vi "Unit Test.vi"() -> ()   [LabVIEW 2018, in "Optris PI.lvlib"]
uses:
  Optris PI/Optris PI.lvlib
  PPLs/Thermal Camera/Parent/Thermal Camera.lvlibp/Accessors/Area Coordinates.ctl
  <vilib>/Utility/miscctls.llb/LVPoint32TypeDef.ctl
  PPLs/Thermal Camera/Parent/Thermal Camera.lvlibp/Thermal Camera.lvclass
panel:
  out "Coords":T1
  out "Area Temps":dbl[][](array[numeric])
  out "Thermal Image":picture
  in  "Path":path=path "C:/RCVR_DATA/RCVRASSET/pic.bmp"
  in  "Cluster":T2={"X"=100, "X Offset"=50, "Y"=100, "Y Offset"=50}
  in  "Min":dbl=-40.0
  in  "Max":dbl=125.0
  in  "Get Thermal Image":bool
  out "error out":errorcluster
  in  "error in (no error)":errorcluster
  in  "Set Temp Range":bool
  in  "Stop":bool
  in  "Connect":bool
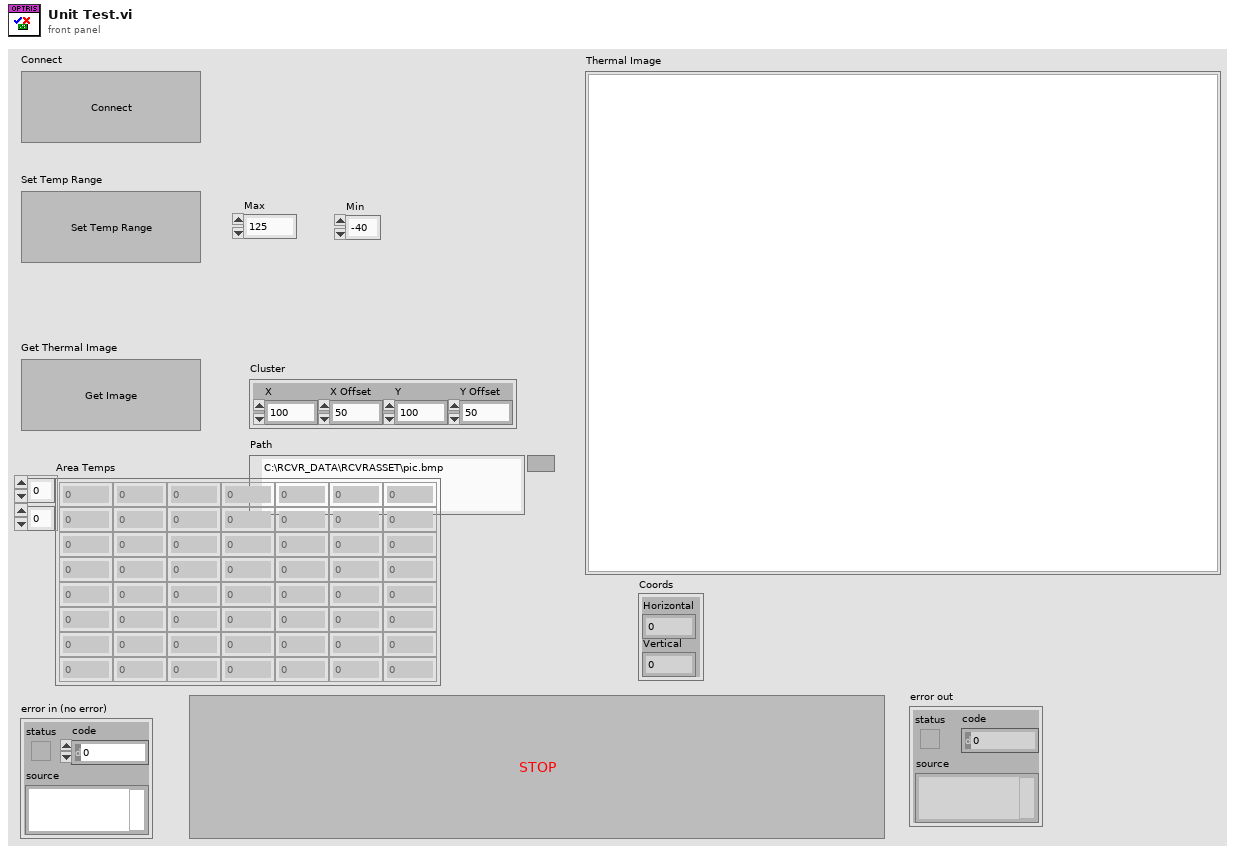
[diagram p1: front panel]
types:
  T1 = typedef "LVPoint32TypeDef.ctl" = cluster{"Horizontal":i32, "Vertical":i32}
  T2 = typedef "Thermal Camera.lvlibp/Thermal Camera.lvclass/Area Coordinates.ctl" = cluster{"X":i32, "X Offset":i32, "Y":i32, "Y Offset":i32}
  T3 = typedef "imagedata.ctl" = cluster{"image type":i32, "image depth":i32, "image":u8[], "mask":u8[], "colors":u32[], "Rectangle":cluster{"left":i16, "top":i16, "right":i16, "bottom":i16}}
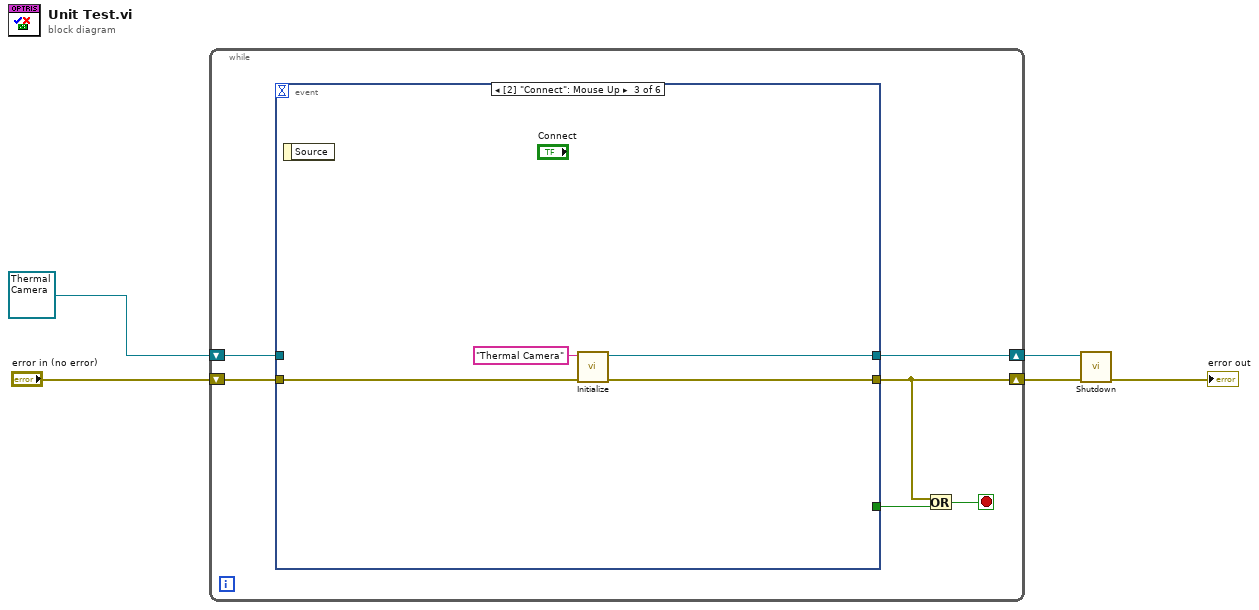
[diagram p0: block diagram]
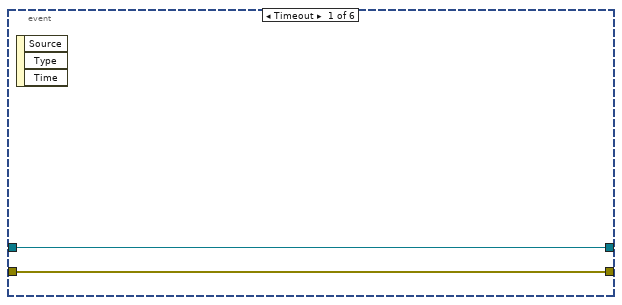
[diagram p2: hidden frame]
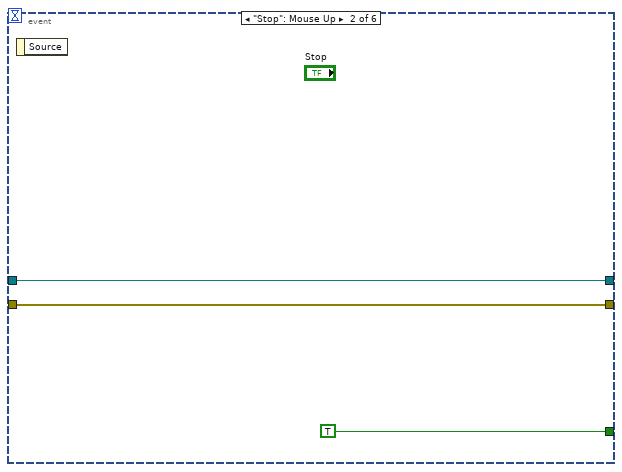
[diagram p3: hidden frame]
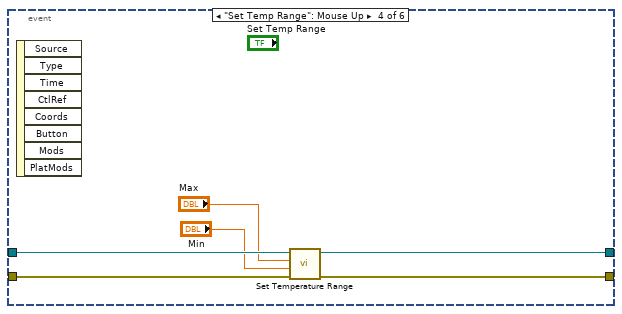
[diagram p4: hidden frame]
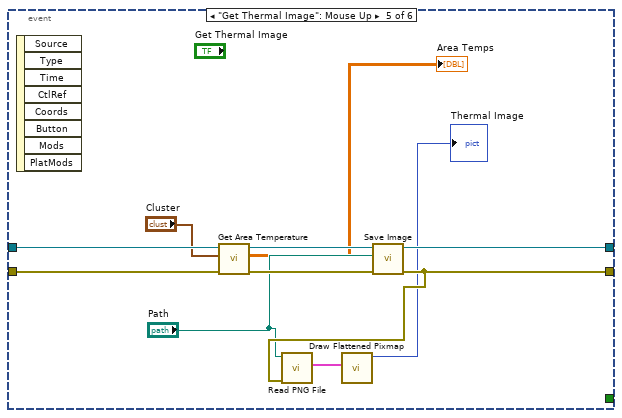
[diagram p5: hidden frame]
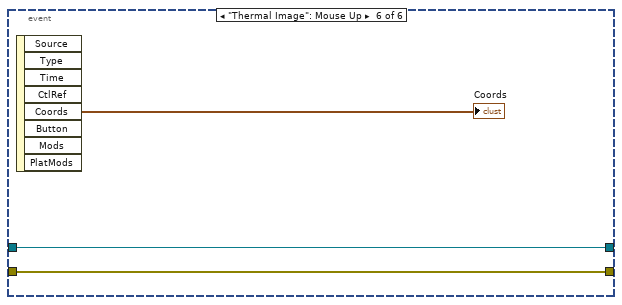
[diagram p6: hidden frame]
diagram:
  n1 = while {
    shift-right: [w7] -> w2
    shift-left: "error in (no error)" -> [w11]
    shift-right: [w10] -> w3
    shift-left: refnum<class "Thermal Camera.lvclass"> refnum ("Thermal Camera out") -> [w9]
    stop <- w6 stop-if-true
    n2 = event shown="[2] \"Connect\": Mouse Up" {
      selector: _ -> [_ _ _ _ _ _]
      dyn-events: _ -> [_ _ _ _ _ _]
      timeout: _ -> [_ _ _ _ _ _]
      tunnel: w11 -> [w12 w15 w20 w25 w36 w38]
      tunnel: [w13 w16 w19 w24 w33 w39] -> w10
      tunnel: [w12 w15 w18 w23 w30 w38] -> w7
      tunnel: w9 -> [w13 w16 _ w26 w37 w39]
      tunnel: [_ TRUE _ _ _ _] -> w8
      event Timeout {
        n3 = event-data() -> ()  [unwired: 1 in, 3 out]
      }
      event "Stop": Mouse Up {
        n4 = event-data() -> ()  [unwired: 1 in, 1 out]
      }
      event "Connect": Mouse Up {
        n5 = event-data() -> ()  [unwired: 1 in, 1 out]
        n6 = call "Initialize.vi"("error in (no error)"=w20, "Name"="Thermal Camera") -> ("error out"=w18:errorcluster, "Thermal Camera out"=w19:refnum<class "Thermal Camera.lvclass">)  [unwired: 8 in]
      }
      event "Set Temp Range": Mouse Up {
        n7 = event-data() -> ()  [unwired: 1 in, 8 out]
        n8 = call-dynamic "Set Temperature Range.vi"("error in (no error)"=w25, "Min"="Min", "Max"="Max", "Thermal Camera in"=w26) -> ("error out"=w23:errorcluster, "Thermal Camera out"=w24:refnum<class "Thermal Camera.lvclass">)  [unwired: 6 in]
      }
      event "Get Thermal Image": Mouse Up {
        n9 = event-data() -> ()  [unwired: 1 in, 8 out]
        n10 = call-dynamic "Get Area Temperature.vi"("error in (no error)"=w36, "Cluster"="Cluster", "Thermal Camera in"=w37) -> ("error out"=w34:errorcluster, "Area Temps"=→"Area Temps":dbl[][], "Thermal Camera out"=w35:refnum<class "Thermal Camera.lvclass">)  [unwired: 5 in, 1 out]
        n11 = call-dynamic "Save Image.vi"("error in (no error)"=w34, "Path"="Path", "Thermal Camera in"=w35) -> ("error out"=w30:errorcluster, "Thermal Camera out"=w33:refnum<class "Thermal Camera.lvclass">)  [unwired: 7 in]
        n12 = call <vilib>:"Read PNG File.vi"("error in (no error)"=w30, "path to PNG file"="Path") -> ("image data"=w31:T3)  [unwired: 7 in, 2 out]
        n13 = call <vilib>:"Draw Flattened Pixmap.vi"("image data"=w31) -> ("new picture"=→"Thermal Image":picture)  [unwired: 8 in]
      }
      event "Thermal Image": Mouse Up {
        n14 = event-data() -> ("Coords"=→"Coords":T1)  [unwired: 1 in, 7 out]
      }
    }
    n15 = Or(x=w7, y=w8) -> (x .or. y?=w6:bool)
  }
  n16 = call "Shutdown.vi"("error in (no error)"=w2, "Thermal Camera in"=w3) -> ("error out"=→"error out":errorcluster)  [unwired: 8 in, 1 out]
